vi "filter pipe - plot staff - more.vi"(0 "omega  in":dbl[](array[numeric]), 1 "zin":cdb[](array[numeric]), 2 "dz/domega in":cdb[](array[numeric]), 3 "z out":cdb[](array[numeric]), 4 "win omega":dbl[](array[numeric]), 5 "phase":dbl[](array[numeric]), 7 "tale of three indices -- int -- control":T1={"left"=0, "center"=0, "right"=0, "right most"=0, "left most"=0, "window"=0, "max win factor"=2, "max win"=2, "min win"=2}, 8 "center":cdb, 9 "Plot: complex plane - filter":refnum<vi>, 11 "Plot: dz/domega":refnum<vi>, 12 "norm":dbl, 13 "Plot: fragment":refnum<vi>, 14 "smart filter: span":dbl(slide)=0.1 min=0.0001 max=0.5 step=0.001 scale=0.001..0.5 scale format="%#_2g", 15 "Plot: win omega":refnum<vi>, 17 "Plot: phase":refnum<vi>) -> ()   [LabVIEW 2010]
uses:
  tale of three indices -- int -- control.ctl
  generate linear region.vi
panel:
  out "size(s) 2":i32
  out "size(s)":i32
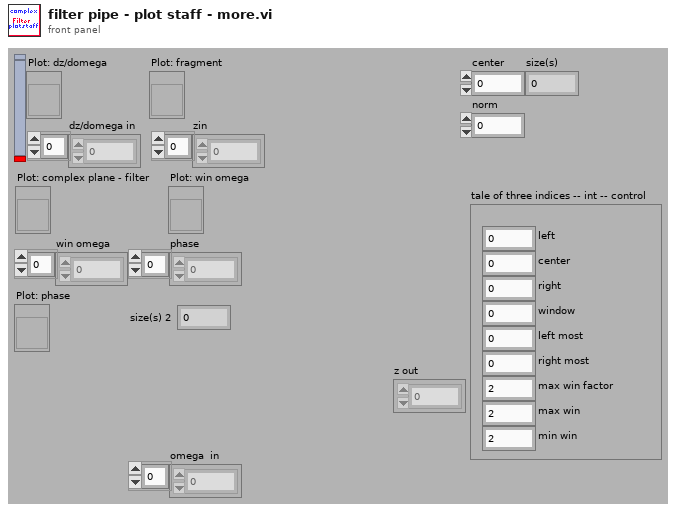
[diagram p1: front panel]
types:
  T1 = typedef "tale of three indices -- int -- control.ctl" = cluster{"left":i32, "center":i32, "right":i32, "right most":i32, "left most":i32, "window":i32, "max win factor":i32, "max win":i32, "min win":i32}
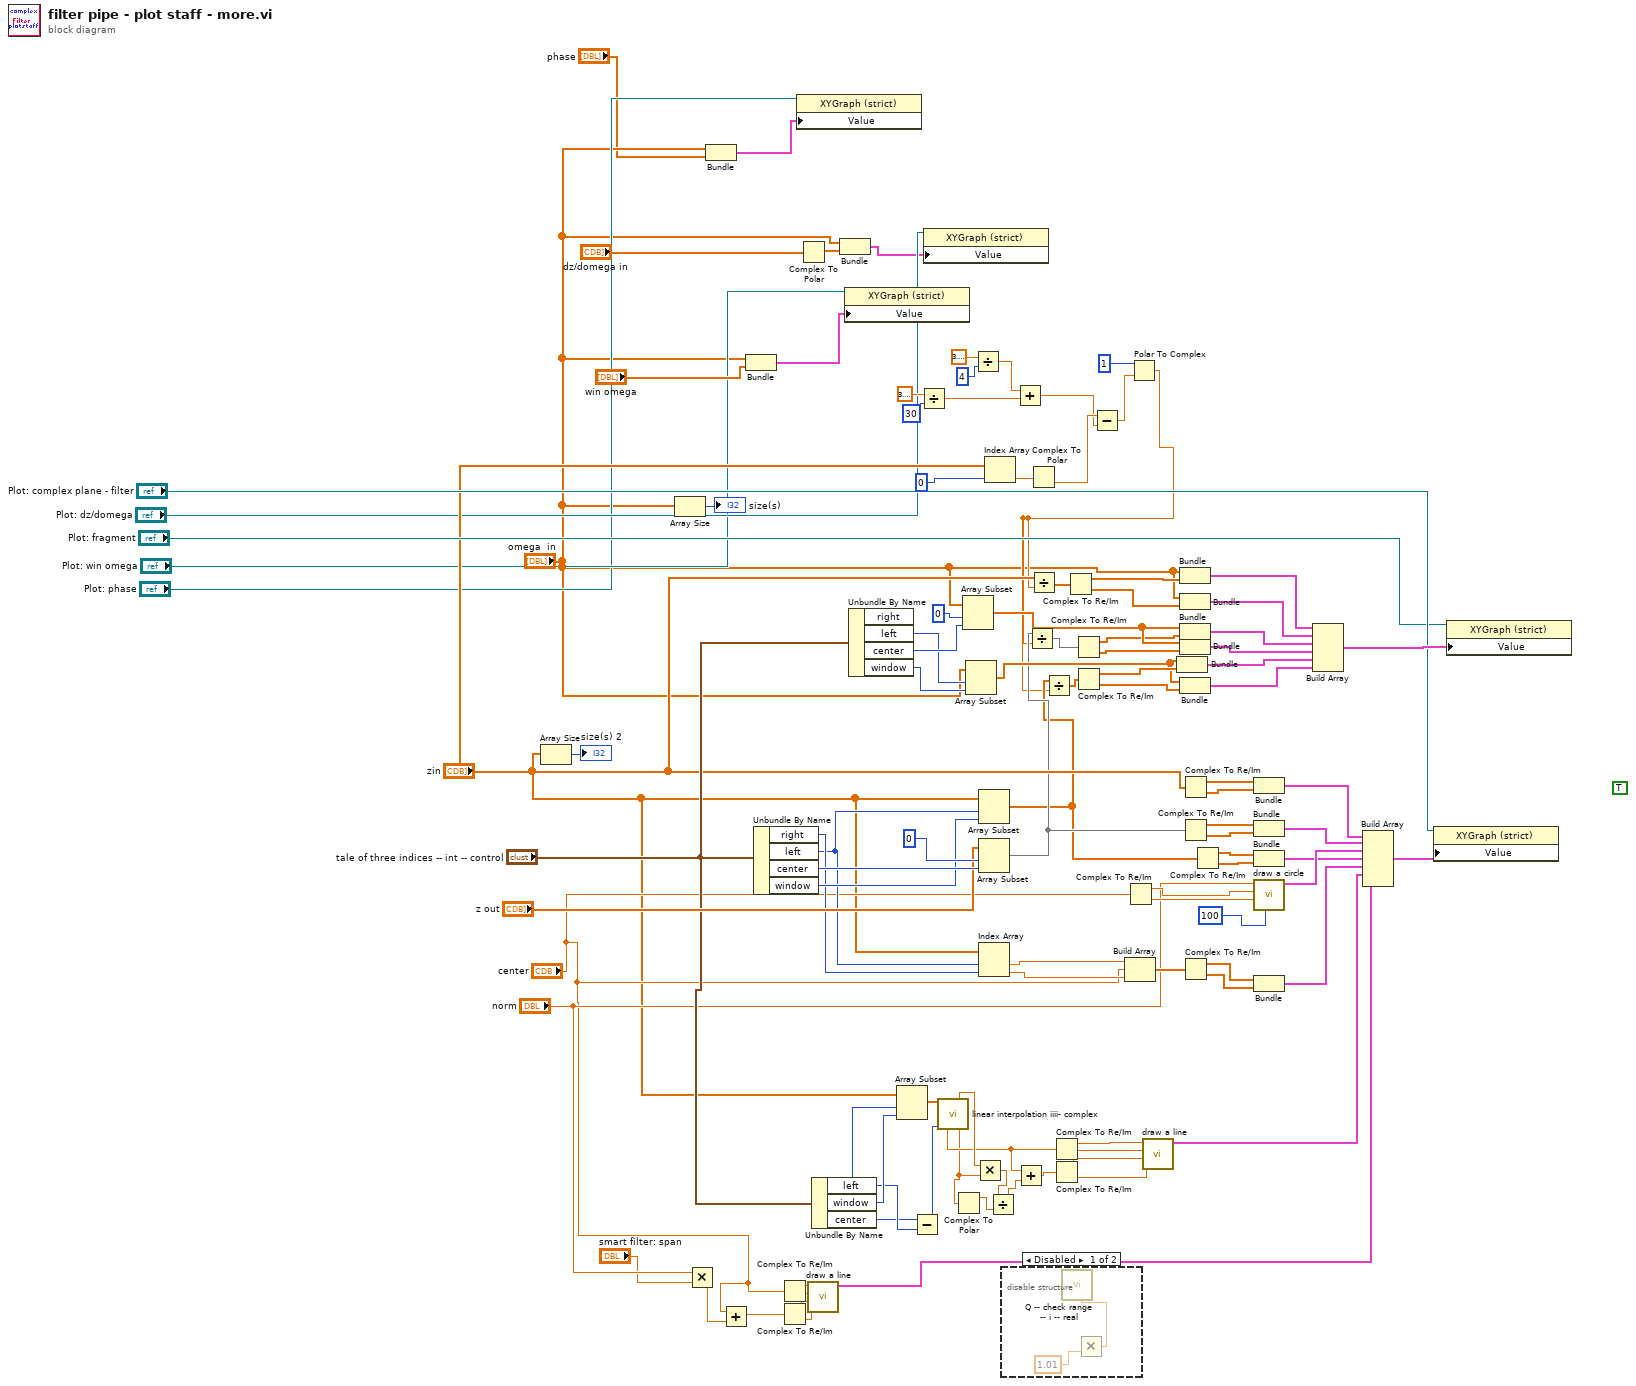
[diagram p0: block diagram]
diagram:
  (unwired) TRUE
  n1 = Array Size(array="zin") -> (size(s)=→"size(s) 2":i32)
  n2 = Array Size(array="omega  in") -> (size(s)=→"size(s)":i32)
  n3 = Multiply(x="norm", y="smart filter: span") -> (x*y=w33:dbl)
  n4 = Bundle("omega  in"="omega  in", "phase"="phase") -> (w3:cluster{"omega  in":dbl[], "phase":dbl[]})  [unwired: 1 in]
  n5 = Add(x="center", y=w33) -> (x+y=w32:cdb)
  n6 = Bundle("omega  in"="omega  in", "win omega"="win omega") -> (w6:cluster{"omega  in":dbl[], "win omega":dbl[]})  [unwired: 1 in]
  n7 = Unbundle By Name("tale of three indices -- int -- control") -> ("right"=w63:i32, "left"=w59:i32, "center"=w68:i32, "window"=w64:i32)
  n8 = Complex To Re/Im(x + iy="center") -> (x=w38:dbl, y=w35:dbl)
  n9 = Complex To Re/Im(x + iy=w32) -> (x=w36:dbl, y=w37:dbl)
  n10 = property class="XYGraph (strict)"(reference="Plot: phase", "Value"=w3) -> ()  [unwired: 1 in, 2 out]
  n11 = Complex To Polar(r * e^(i*theta)="dz/domega in") -> (r=w11:dbl[])  [unwired: 1 out]
  n12 = call "draw a line.vi"("y1"=w37, "y0"=w35, "x1"=w36, "x0"=w38) -> ("output cluster"=w31:cluster{dbl[], dbl[]})  [unwired: 7 in]
  n13 = Unbundle By Name("tale of three indices -- int -- control") -> ("left"=w56:i32, "window"=w57:i32, "center"=w55:i32)
  n14 = Bundle("omega  in"="omega  in", w11) -> (w8:cluster{"omega  in":dbl[], dbl[]})  [unwired: 1 in]
  n15 = property class="XYGraph (strict)"(reference="Plot: win omega", "Value"=w6) -> ()  [unwired: 1 in, 2 out]
  n16 = Unbundle By Name("tale of three indices -- int -- control") -> ("left"=w82:i32, "center"=w84:i32, "window"=w81:i32)  [unwired: 1 out]
  n17 = Array Subset(array="zin", index=w56, length=w57) -> (w58:cdb[])
  n18 = Subtract(x=w55, y=w56) -> (x-y=w54:i32)
  n19 = Divide(x=3.141592653589793, y=30) -> (x/y=w12:dbl)
  n20 = property class="XYGraph (strict)"(reference="Plot: dz/domega", "Value"=w8) -> ()  [unwired: 1 in, 2 out]
  n21 = call "linear interpolation iiii- complex.vi"("Array"=w58, "center"=w54) -> ("directed sigma"=w51:dbl, "intercept"=w50:cdb, "slope"=w44:cdb)  [unwired: 5 in, 6 out]
  n22 = Complex To Polar(r * e^(i*theta)=w44) -> (r=w43:dbl)  [unwired: 1 out]
  n23 = Array Subset(array="omega  in", index=0, length=w84) -> (w83:dbl[])
  n24 = Array Subset(array="omega  in", index=w82, length=w81) -> (w72:dbl[])
  n25 = Divide(x=3.141592653589793, y=4) -> (x/y=w16:dbl)
  n26 = Multiply(x=w51, y=w44) -> (x*y=w42:cdb)
  n27 = Array Subset(array="zin", index=w59, length=w64) -> (w24:cdb[])
  n28 = Array Subset(array="z out", index=0, length=w68) -> (w26:cdb[])
  n29 = Index Array(array="zin", index #1=w59, index #2=w63) -> (element #1=w66:cdb, element #2=w65:cdb)
  n30 = Index Array(array="zin", index=0) -> (element=w28:cdb)
  n31 = Divide(x=w42, y=w43) -> (x/y=w41:cdb)
  n32 = disable-structure shown="Disabled" {
    frame Disabled {
      n33 = Multiply(y=1.01) -> (x*y=w108:dbl)  [unwired: 1 in]
      n34 = call "Q -- check range -- i -- real.vi"("upper"=w108) -> ()  [unwired: 8 in, 3 out]
    }
    frame Enabled {
    }
  }
  n35 = Add(x=w16, y=w12) -> (x+y=w15:dbl)
  n36 = Add(x=w50, y=w41) -> (x+y=w49:cdb)
  n37 = Complex To Polar(r * e^(i*theta)=w28) -> (theta=w19:dbl)  [unwired: 1 out]
  n38 = Complex To Re/Im(x + iy=w50) -> (x=w52:dbl, y=w45:dbl)
  n39 = Complex To Re/Im(x + iy=w49) -> (x=w46:dbl, y=w48:dbl)
  n40 = Subtract(x=w19, y=w15) -> (x-y=w18:dbl)
  n41 = Build Array(w66, "center", w65) -> (w62:cdb[])
  n42 = Complex To Re/Im(x + iy="center") -> (x=w101:dbl, y=w100:dbl)
  n43 = Polar To Complex(1:w18, 2:1) -> (0:w17:cdb)
  n44 = Divide(x=w26, y=w17) -> (x/y=w25:cdb[])
  n45 = Divide(x="zin", y=w17) -> (x/y=w27:cdb[])
  n46 = Divide(x=w24, y=w17) -> (x/y=w23:cdb[])
  n47 = Complex To Re/Im(x + iy=w27) -> (x=w88:dbl[], y=w87:dbl[])
  n48 = Complex To Re/Im(x + iy=w25) -> (x=w78:dbl[], y=w77:dbl[])
  n49 = Complex To Re/Im(x + iy=w23) -> (x=w74:dbl[], y=w73:dbl[])
  n50 = call "draw a line.vi"("y1"=w48, "y0"=w45, "x1"=w46, "x0"=w52) -> ("output cluster"=w47:cluster{dbl[], dbl[]})  [unwired: 7 in]
  n51 = Bundle(w72, w74) -> (w71:cluster{dbl[], dbl[]})  [unwired: 1 in]
  n52 = Bundle("omega  in"="omega  in", w88) -> (w86:cluster{"omega  in":dbl[], dbl[]})  [unwired: 1 in]
  n53 = Bundle("omega  in"="omega  in", w87) -> (w90:cluster{"omega  in":dbl[], dbl[]})  [unwired: 1 in]
  n54 = Bundle(w83, w78) -> (w76:cluster{dbl[], dbl[]})  [unwired: 1 in]
  n55 = Bundle(w83, w77) -> (w75:cluster{dbl[], dbl[]})  [unwired: 1 in]
  n56 = Bundle(w72, w73) -> (w70:cluster{dbl[], dbl[]})  [unwired: 1 in]
  n57 = Complex To Re/Im(x + iy="zin") -> (x=w107:dbl[], y=w106:dbl[])
  n58 = Complex To Re/Im(x + iy=w26) -> (x=w105:dbl[], y=w104:dbl[])
  n59 = Complex To Re/Im(x + iy=w62) -> (x=w93:dbl[], y=w92:dbl[])
  n60 = Complex To Re/Im(x + iy=w24) -> (x=w96:dbl[], y=w95:dbl[])
  n61 = Bundle(w107, w106) -> (w103:cluster{dbl[], dbl[]})  [unwired: 1 in]
  n62 = Bundle(w105, w104) -> (w102:cluster{dbl[], dbl[]})  [unwired: 1 in]
  n63 = Bundle(w96, w95) -> (w94:cluster{dbl[], dbl[]})  [unwired: 1 in]
  n64 = call "draw a circle.vi"("number of points"=100, "center Y"=w100, "center x"=w101, "radius"="norm") -> ("output cluster"=w98:cluster{dbl[], dbl[]})  [unwired: 7 in]
  n65 = Bundle(w93, w92) -> (w91:cluster{dbl[], dbl[]})  [unwired: 1 in]
  n66 = Build Array(w86, w90, w76, w75, w71, w70) -> (w89:cluster{"omega  in":dbl[], dbl[]}[])
  n67 = Build Array(w103, w102, w98, w94, w91, w47, w31) -> (w97:cluster{dbl[], dbl[]}[])
  n68 = property class="XYGraph (strict)"(reference="Plot: complex plane - filter", "Value"=w97) -> ()  [unwired: 1 in, 2 out]
  n69 = property class="XYGraph (strict)"(reference="Plot: fragment", "Value"=w89) -> ()  [unwired: 1 in, 2 out]
